vi "DeviceNameTCPWrite.vi"(8 "error in (no error)":errorcluster, 11 "connection ID":refnum<k5>) -> (0 "error out":errorcluster, 3 "connection ID out":refnum<k5>)   [LabVIEW 2020]
panel:
  out "Reply String":string
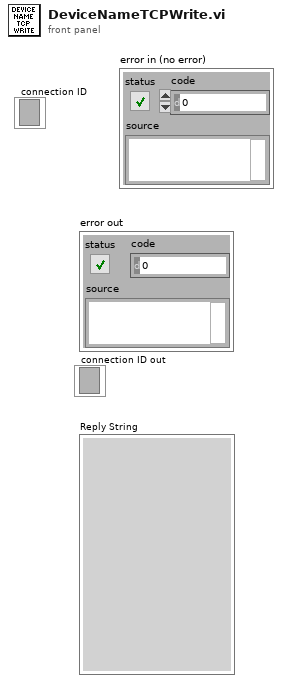
[diagram p1: front panel]
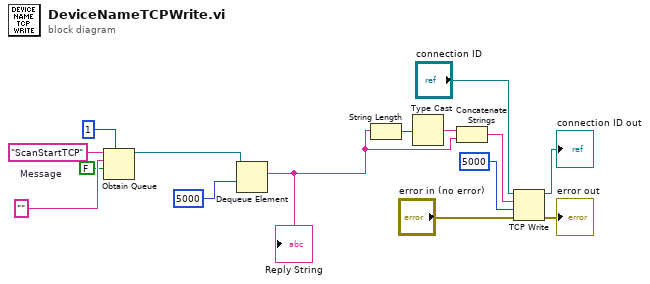
[diagram p0: block diagram]
diagram:
  w7 = ""  # Message
  n1 = Obtain Queue(max queue size (-1, unlimited)=1, name (unnamed)="ScanStartTCP", element data type=w7, create if not found? (T)=FALSE) -> (queue out=w3:refnum<queue>)  [unwired: 1 in, 2 out]
  n2 = Dequeue Element(queue=w3, timeout in ms (-1)=5000) -> (element=w1:string)  [unwired: 1 in, 3 out]
  "Reply String" <- w1
  n3 = String Length(string=w1) -> (length=w13:i32)
  n4 = Type Cast(x=w13) -> (*(type *) &x=w12:string)  [unwired: 1 in]
  n5 = Concatenate Strings(w12, w1) -> (w11:string)
  n6 = TCP Write(connection ID="connection ID", data in=w11, error in (no error)="error in (no error)", 9:5000 ("timeout ms (25000)")) -> (connection ID out=→"connection ID out":refnum<k5>, error out=→"error out":errorcluster)  [unwired: 1 out]
